vi "ErrorCodeToErrorStringConverter.vi"(8 "error in (no error)":errorcluster, 11 "StatusInfo":T1) -> (0 "error out":errorcluster)   [LabVIEW 2017, in "fgt_SDK.lvlib"]
uses:
  fgt_SDK.lvlib
  TypeDefs/fgt_STATUS_INFO.ctl
  TypeDefs/fgt_INSTRUMENT_TYPE.ctl
  TypeDefs/fgt_ERROR_CODE.ctl
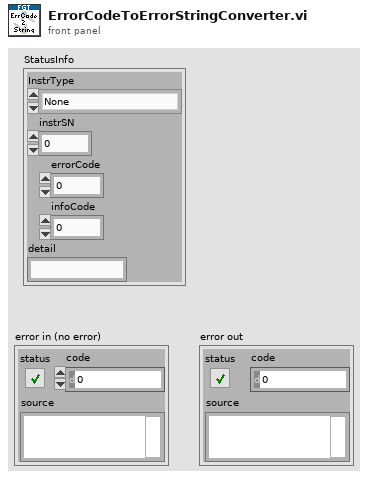
[diagram p1: front panel]
types:
  T1 = typedef "fgt_SDK.lvlib/fgt_STATUS_INFO.ctl" = cluster{"InstrType":T2, "instrSN":u16, "errorCode":u8, "infoCode":u8, "detail":string}
  T2 = typedef "fgt_SDK.lvlib/fgt_INSTRUMENT_TYPE.ctl" = enum32{"None", "MFCS", "MFCS_EZ", "FRP", "LineUP", "IPS"}
  T3 = typedef "fgt_SDK.lvlib/fgt_ERROR_CODE.ctl" = enum8{"OK", "USB_error", "Wrong_command", "No_Module_at_index", "Wrong_module", "Module_is_sleep", "Master_error", "Failed_init_all_instr", "Wrong_parameter", "Overpressure", "Underpressure", "No_instr_found", "No_modules_found", "No_pressure_controller_found", "Dll_dependency_error"}
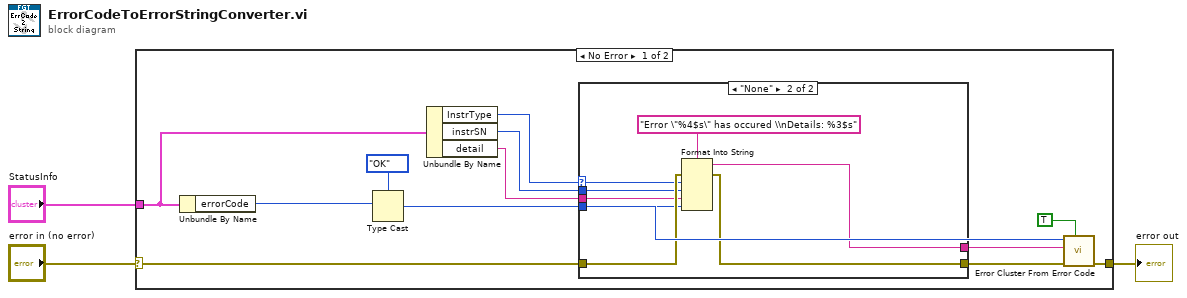
[diagram p0: block diagram]
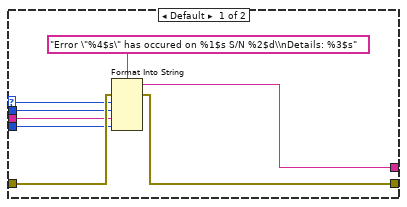
[diagram p2: hidden frame]
diagram:
  n1 = case shown="No Error" "error in (no error)" {
    selector: "error in (no error)" -> [w14 w32]
    tunnel: [w15 w32] -> w3
    tunnel: "StatusInfo" -> [w11 _]
    frame No Error {
      n2 = Unbundle By Name(w11) -> ("errorCode"=w4:u8)
      n3 = Type Cast(type=fgt_ERROR_CODE."OK" ("fgt_ERROR_CODE"), x=w4) -> (*(type *) &x=w12:T3)
      n4 = Unbundle By Name(w11) -> ("InstrType"=w9:T2, "instrSN"=w8:u16, "detail"=w7:string)
      n5 = case shown="\"None\"" w9 {
        selector: w9 -> [w21 w29]
        tunnel: w14 -> [w23 w31]
        tunnel: w12 -> [w22 w30]
        tunnel: w8 -> [w20 w28]
        tunnel: w7 -> [w19 w27]
        tunnel: [w18 w26] -> w6
        tunnel: [w16 w24] -> w5
        frame Default {
          n6 = Format Into String(format string="Error \"%4$s\" has occured on %1$s S/N %2$d\\nDetails: %3$s", error in=w23, w21, w20, w19, w22) -> (resulting string=w16:string, error out=w18:errorcluster)  [unwired: 1 in]
        }
        frame "None" {
          n7 = Format Into String(format string="Error \"%4$s\" has occured \\nDetails: %3$s", error in=w31, w29, w28, w27, w30) -> (resulting string=w24:string, error out=w26:errorcluster)  [unwired: 1 in]
        }
      }
      n8 = call <vilib>:"Error Cluster From Error Code.vi"("show call chain? (False)"=TRUE, "error in (no error)"=w6, "error message (\"\")"=w5, "error code (0)"=w12) -> ("error out"=w15:errorcluster)  [unwired: 5 in]
    }
    frame Error {
    }
  }
  "error out" <- w3
